vi "Alpha Ver 1.2.vi"() -> ()   [LabVIEW 2015]
uses:
  <instrlib>/Keithley 622x LV 2009/Configure/Source/Typedefs/KE622x -- Current Range.ctl
  <instrlib>/Keithley 622x LV 2009/Configure/Source/Typedefs/KE622x -- Current Ranges.ctl
  <instrlib>/Keithley 622x LV 2009/Typedefs/KE622x -- On Off Control.ctl
  <instrlib>/Keithley 622x LV 2009/Utility/Typedefs/KE622x -- Instrument Type.ctl
  <instrlib>/Keithley 622x LV 2009/Configure/Source/Typedefs/KE622x -- Voltage Limit.ctl
  <instrlib>/Keithley 2000/Public/Configure/Configure DC Volts.vi
  <userlib>/LV-Link3/PolySubVIs/DtCreateAinChan.vi
  <userlib>/LV-Link3/PolySubVIs/DtOLReadMultipleSingle.vi
  <instrlib>/Keithley 2000/Keithley 2000.lvlib
  <instrlib>/Keithley 622x LV 2009/Keithley 622x.lvlib
panel:
  out "DAQ A4":dbl format="%#_13g"
  out "DAQ_clust":T1
  out "DAQ A3":dbl format="%#_13g"
  out "DAQ A2":dbl format="%#_13g"
  out "DAQ A1":dbl format="%#_13g"
  out "Real stop cur":dbl format="%#_13g"
  out "Real start cur":dbl format="%#_13g"
  in  "Stop cur prefix":u16(ring)=2
  in  "Start cur prefix":u16(ring)=2
  out "MULTIPLE GRAPHS":cluster{dbl[], dbl[]}[](graph)
  in  "X-Axis":T2(ring)
  in  "Range":u8(ring)=20 items=["100nV", "200nV", "500nV", "1µV", "2µV", "5µV", "10µV", "20µV", "50µV", "100µV", "200µV", "500µV", "1mV", "2mV", "5mV", "10mV", "20mV", "50mV", "100mV", "200mV", "500mV", "1V"]
  in  "Display Type copy":u16(ring)=3 items=["X %", "Y %", "X Calibrated", "Y Calibrated", "Mag %", "Mag Calibrated", "Phase Degrees", "Ratio", "ADC 1", "ADC 2", "ADC 3", "ADC 4 ", "Noise %", "Noise Calibrated", "Ref Frequency", "", ""]
  out "Units copy":string
  out "Display copy":dbl format="%.3f"
  out "Overload":bool
  out "Display":dbl format="%.3f"
  out "Units":string
  in  "Display Type":u16(ring)=2 items=["X %", "Y %", "X Calibrated", "Y Calibrated", "Mag %", "Mag Calibrated", "Phase Degrees", "Ratio", "ADC 1", "ADC 2", "ADC 3", "ADC 4 ", "Noise %", "Noise Calibrated", "Ref Frequency", "", ""]
  in  "Time Constant":u16(ring) items=["MIN", "1ms", "3ms", "10ms", "30ms", "100ms", "300ms", "1s", "3s", "10s", "30s", "100s", "300s"]
  in  "Slope":u8(ring) items=["6db/octave", "12dB/octave"]
  in  "Dynamic Reserve":u16(ring) items=["High Stability", "Normal", "High Reserve"]
  in  "Auto Sensitivity":bool
  in  "Auto Measure":bool
  out "6221_error_out":errorcluster
  out "2000_error_out":errorcluster
  out "5110_error_out":errorcluster
  out "Input Mode":i32(ring) items=[" Voltage Input (A or A-B) ", "Current Input 10E6 V/A", "Current Input 10E8 V/A"]
  out "5110":refnum<visa-resource-name>
  in  "GPIB Address":i8=11 min=1 max=32 step=1
  out "DAQ A0":dbl format="%#_13g"
  out "2000":dbl format="%#_13g"
  in  "Device":string(combo)
  in  "Number \nof points":i32
  in  "Folder\nprename":string
  out "TIME GRAPH":cluster{dbl[], dbl[]}[](graph)
  out "T0":u32
  out "LIMIT":bool
  out "LIMIT":bool
  out "Error Code":string
  in  "Comments":string
  out "file":refnum<file>
  out "2000":refnum<visa-resource-name>
  out "6221":refnum<visa-resource-name>
  out "Step  (A)":dbl=5e-05 format="%#_3p"
  in  "Stop\ncurrent (A)":dbl=2.0 format="%#_6p"
  in  "Start \ncurrent (A)":dbl=1.0 format="%#_6p"
  in  "Check For SCPI Errors? (T)":bool=TRUE
  out "Interlock Tripped?":bool
  out "Compliance?":bool
  in  "Turn Off Output \nIf Compliance?":bool=TRUE
  in  "Turning ON/OFF\ncurrent output":T3=enum."On"
  in  "Range Selection":T4={"Auto Range?"=TRUE, "Man / Selected\nRange"=enum."2nA"}
  # "FILE CONFIGURATION"
  # "ADMIN PANEL"
  # "KEITHLEY 6221 CONFIGURATION (ADMIN ONLY)"
  # "KEITHLEY DAQ CONFIGURATION (ADMIN ONLY)"
  # "PRINCETON LOCK-IN AMP (ADMIN ONLY)"
  # "I don't know what the hell it is,\njust don't touch it"
  # "SENSITIVITY"
  # "INPUT CONFIGURATION"
  # "READINGS"
  # "START, STOP, STEP, CONFIGURATION"
  # "IF ON"
  # "Output Channels Time - Constant \nSlope & Dynamic Reserve"
  # "Compliance = Limiting output voltage\nThis switch determines if we want to switch \noff the current output if wee exceed compliance"
  # "LOCK-IN READINGS"
  # "RIGHT DISPLAY"
  # "LEFT DISPLAY"
  # "There is a safe switch at \nthe back of the instrument \nThis indicator shows if it is on"
  # "You have hit a damn jackpot \nby exceeding the limited voltage\nCongrats"
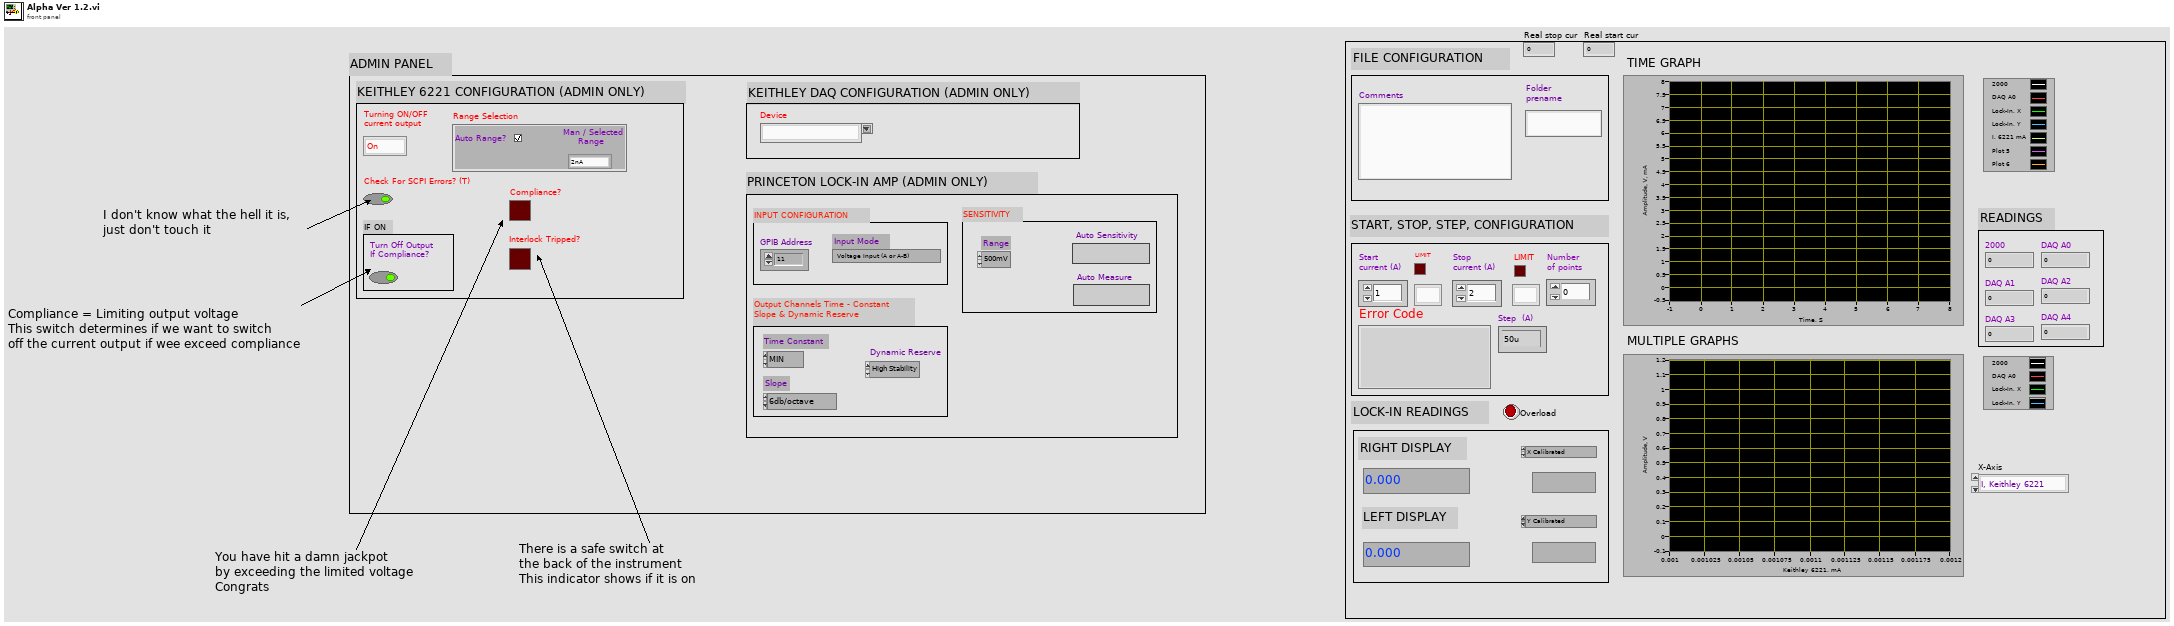
[diagram p1: front panel]
types:
  T1 = cluster{"Task out":i32, "Actual Number of Channels":u32, "error out":errorcluster}
  T2 = enum16{"I, Keithley 6221", "V, Keithley 2000", "V, Keithley DAQ A0", "V, Keithley DAQ A1", "V, Keithley DAQ A2", "V, Keithley DAQ A3", "V, Keithley DAQ A4", "V, Lock-In X", "V, Lock-In Y"}
  T3 = typedef "Keithley 622x.lvlib/KE622x -- On Off Control.ctl" = enum16{"Off", "On"}
  T4 = typedef "Keithley 622x.lvlib/KE622x -- Current Range.ctl" = cluster{"Auto Range?":bool, "Man / Selected\nRange":T5}
  T5 = typedef "Keithley 622x.lvlib/KE622x -- Current Ranges.ctl" = enum16{"2nA", "20nA", "200nA", "2uA", "20uA", "200uA", "2mA", "20mA", "100mA"}
  T6 = typedef "Keithley 622x.lvlib/KE622x -- Instrument Type.ctl" = enum16{"KE6220", "KE6221"}
  T7 = typedef "Keithley 622x.lvlib/KE622x -- Voltage Limit.ctl" = dbl
  T8 = cluster{"Task out":i32, "error out":errorcluster}
  T9 = cluster{dbl, dbl, dbl, dbl, dbl, "Measurement":dbl}
  T10 = cluster{dbl[], dbl[], dbl[], dbl[], dbl[], dbl[], dbl[], dbl[], dbl[], dbl[]}
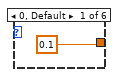
[diagram p2: hidden frame]
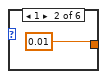
[diagram p3: hidden frame]
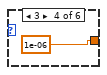
[diagram p4: hidden frame]
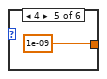
[diagram p5: hidden frame]
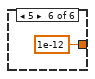
[diagram p6: hidden frame]
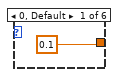
[diagram p7: hidden frame]
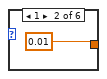
[diagram p8: hidden frame]
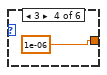
[diagram p9: hidden frame]
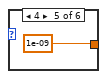
[diagram p10: hidden frame]
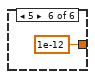
[diagram p11: hidden frame]
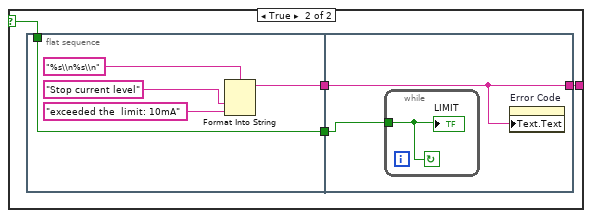
[diagram p12: hidden frame]
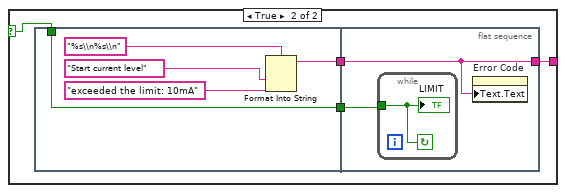
[diagram p13: hidden frame]
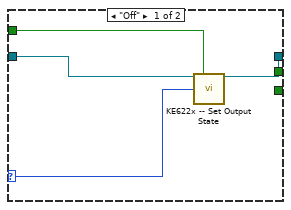
[diagram p14: hidden frame]
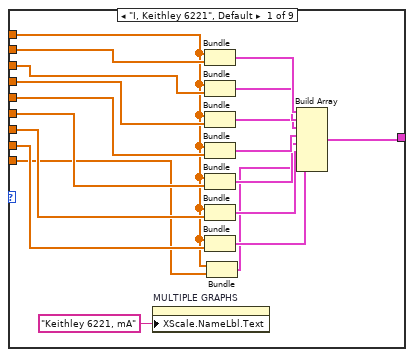
[diagram p15: hidden frame]
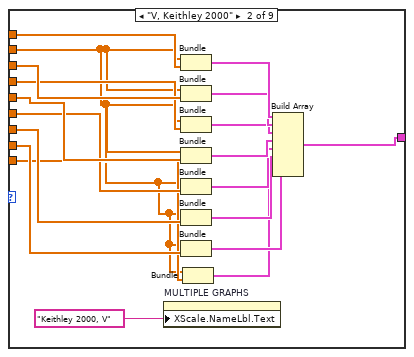
[diagram p16: hidden frame]
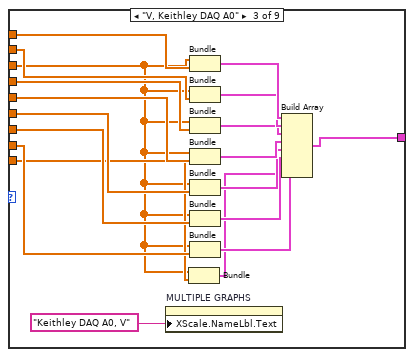
[diagram p17: hidden frame]
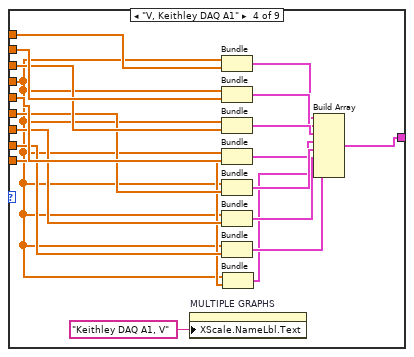
[diagram p18: hidden frame]
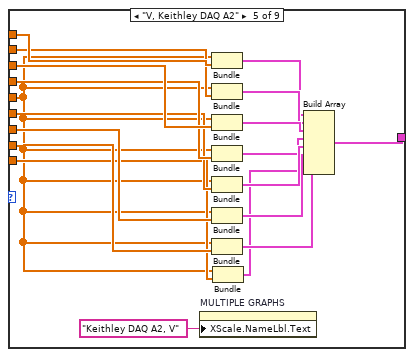
[diagram p19: hidden frame]
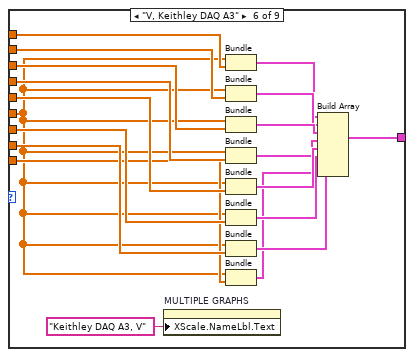
[diagram p20: hidden frame]
diagram:
  n1 = flat-sequence {
    tunnel: [w175] -> w7
    tunnel: [w174] -> w6
    tunnel: [w173] -> w5
    tunnel: [w172] -> w4
    tunnel: [w171] -> w3
    tunnel: [w170] -> w2
    tunnel: [w159] -> w1
    tunnel: w7 -> [w800]
    tunnel: w6 -> [w799]
    tunnel: w5 -> [w798]
    tunnel: w4 -> [w797]
    tunnel: w3 -> [w796]
    tunnel: w2 -> [w795]
    tunnel: w1 -> [w794]
    frame #0 {
      # "File configuration"
      # "Start, Stop, Step"
      # "Time Intit"
      # "Initializing instruments"
      n2 = flat-sequence {
        frame #0 {
          w16 = TRUE  # reset
          w15 = FALSE  # ID query
          # "Initialize Lock-In 5110"
          # "Initialize Keithley 2000"
          # "Initialize Keithley 6221"
          n3 = call <instrlib>:"Initialize.vi"("VISA resource name"=refnum<visa-resource-name> "KEITHLEY_MULTIMETER") -> ("VISA resource name out"=w20:refnum<visa-resource-name>)  [unwired: 17 in, 1 out]
          n4 = call <instrlib>:"Initialize.vi"("VISA resource name"=refnum<visa-resource-name> "KEITHLEY_DC_AC_CURRENT_SOURCE", "Error Queue Option"=enum16{"Clear Error Queue", "Error Query"}."Clear Error Queue", "Instrument Type"=KE622x_--_Instrument_Type."KE6221") -> ("VISA resource name out"=→"6221":refnum<visa-resource-name>, "error out"=→"6221_error_out":errorcluster)  [unwired: 11 in]
          n5 = call "SR51XX Initialize"("VISA session (for class)"=refnum<visa-resource-name> "LOCK_IN_5110_PRINCETON", "Interface"=FALSE, "ID query"=w15, "GPIB Address"="GPIB Address", "reset"=w16) -> ("VISA session"=→"5110":refnum<visa-resource-name>, "error out"=→"5110_error_out":errorcluster)  [unwired: 8 in, 1 out]
          n6 = call-poly <instrlib>:"Configure Measurement.vi"("VISA resource name"=w20) -> ("VISA resource name out"=→"2000":refnum<visa-resource-name>, "error out"=→"2000_error_out":errorcluster)  [unwired: 17 in]
        }
        frame #1 {
          # "Initialize Keithley DAQ \n(getting board name)"
          n7 = call <userlib>:"DtOLGetBoardNames.vi"() -> ("Number of boards"=w25:u32)  [unwired: 9 in, 2 out]
          n8 = Initialize Array("", w25) -> (w27:string[])
          n9 = for {
            N: w25 -> [_]
            shift-right: [w33] -> w30
            shift-left: w27 -> [w34]
            i -> [w32]
            n10 = Add(x=1, y=w32) -> (x+y=w36:i32)
            n11 = call <userlib>:"DtOLGetBoardNames.vi"("Select Board"=w36) -> ("Board Name"=w31:string)  [unwired: 8 in, 2 out]
            n12 = Replace Array Subset(array=w34, new element=w31, index=w32) -> (w33:string[])
          }
          n13 = Index Array(array=w30, index=0) -> (element=w29:string)
          n14 = property on="Device" class="CmbBox"("Strings[]"=w30, "Value"=w29) -> ()  [unwired: 2 in, 2 out]
        }
        frame #2 {
          # "Calculating steps by number\nof points"
          # "Putting in a loop \ninstead of \"STOP\""
          n15 = local read "Real stop cur"() -> (w53:dbl)
          n16 = local read "Real start cur"() -> (w54:dbl)
          n17 = case shown="2" "Start cur prefix" {
            tunnel: [0.1 0.01 0.001 1e-06 1e-09 1e-12] -> w42
            frame 0, Default {
            }
            frame 1 {
            }
            frame 2 {
            }
            frame 3 {
            }
            frame 4 {
            }
            frame 5 {
            }
          }
          n18 = case shown="2" "Stop cur prefix" {
            tunnel: [0.1 0.01 0.001 1e-06 1e-09 1e-12] -> w40
            frame 0, Default {
            }
            frame 1 {
            }
            frame 2 {
            }
            frame 3 {
            }
            frame 4 {
            }
            frame 5 {
            }
          }
          n19 = Subtract(x=w53, y=w54) -> (x-y=w56:dbl)
          n20 = Multiply(x=w42, y="Start \ncurrent (A)") -> (x*y=w38:dbl)
          "Real start cur" <- w38
          n21 = Divide(x=w56, y="Number \nof points") -> (x/y=→"Step  (A)":dbl)
          n22 = Multiply(x=w40, y="Stop\ncurrent (A)") -> (x*y=w37:dbl)
          "Real stop cur" <- w37
          n23 = Greater?(x=w37, y=T7 0.01) -> (0:w48:bool)
          n24 = Greater?(x=w38, y=T7 0.01) -> (0:w47:bool)
          n25 = case shown="False" w48 {
            selector: w48 -> [_ w72]
            tunnel: [w69 w75] -> w50
            frame False {
              n26 = Format Into String(format string="%s\\n", "Start current level is OK" ("false string")) -> (resulting string=w69:string)  [unwired: 2 in, 1 out]
            }
            frame True {
              n27 = flat-sequence {
                tunnel: [w77] -> w74
                tunnel: [w76] -> w73
                tunnel: w72 -> [w76]
                tunnel: [w81] -> w75
                tunnel: w74 -> [w81]
                tunnel: w73 -> [w82]
                frame #0 {
                  n28 = Format Into String(format string="%s\\n%s\\n", "Stop current level" ("String"), "exceeded the  limit: 10mA" ("input 2")) -> (resulting string=w77:string)  [unwired: 2 in, 1 out]
                }
                frame #1 {
                  n29 = while {
                    tunnel: w82 -> [w83]
                    stop <- w83 continue-if-true
                    "LIMIT" <- w83
                  }
                  n30 = property on="Error Code" class="Str"("Text.Text"=w81) -> ()  [unwired: 2 in, 2 out]
                }
              }
            }
          }
          n31 = case shown="False" w47 {
            selector: w47 -> [_ w88]
            tunnel: [w84 w90] -> w49
            frame False {
              n32 = Format Into String(format string="%s\\n", "Start current level is OK" ("false string")) -> (resulting string=w84:string)  [unwired: 2 in, 1 out]
            }
            frame True {
              n33 = flat-sequence {
                tunnel: [w92] -> w89
                tunnel: w88 -> [w91]
                tunnel: [w91] -> w87
                tunnel: [w96] -> w90
                tunnel: w89 -> [w96]
                tunnel: w87 -> [w97]
                frame #0 {
                  n34 = Format Into String(format string="%s\\n%s\\n", "Start current level" ("String"), "exceeded the limit: 10mA" ("input 2")) -> (resulting string=w92:string)  [unwired: 2 in, 1 out]
                }
                frame #1 {
                  n35 = while {
                    tunnel: w97 -> [w98]
                    stop <- w98 continue-if-true
                    "LIMIT" <- w98
                  }
                  n36 = property on="Error Code" class="Str"("Text.Text"=w96) -> ()  [unwired: 2 in, 2 out]
                }
              }
            }
          }
          n37 = Concatenate Strings(w49, w50) -> (→"Error Code":string)
        }
        frame #3 {
          n38 = flat-sequence {
            frame #0 {
              # "Creating folder&file"
              n39 = call "folder_creation.vi"("Name"="Folder\nprename") -> ("String"=w100:string)
              n40 = call "file_creation.vi"("String"=w100) -> ("refnum out"=→"file":refnum<file>)
            }
            frame #1 {
              # "Creating comments"
              n41 = local read "file"() -> (w102:refnum<file>)
              n42 = Format Into String(format string="# %s\\n", initial string=w102, "Comments") -> ()  [unwired: 1 in, 2 out]
            }
            frame #2 {
              # "Writing instr params"
              n43 = local read "5110"() -> (w110:refnum<visa-resource-name>)
              n44 = local read "Real stop cur"() -> (w108:dbl)
              n45 = local read "file"() -> (w105:refnum<file>)
              n46 = local read "Real start cur"() -> (w109:dbl)
              n47 = call "com_inst.vi"("Stop current"=w108, "Start current"=w109, "VISA session (for class)"=w110) -> ("concatenated string"=w106:string)
              n48 = Format Into String(format string="# %s\\n", initial string=w105, w106) -> ()  [unwired: 1 in, 2 out]
            }
            frame #3 {
              # "Adding headlines"
              n49 = local read "file"() -> (w122:refnum<file>)
              n50 = Format Into String(format string="# %-6s  %-12s %-12s %-14s %-12s %-14s %-12s %-14s %-14s%-14s\\n", initial string=w122, "t, ms" ("input 3"), "2000, V" ("input 1"), "DAQ A0, V" ("input 2"), "DAQ A1, V" ("input 2"), "DAQ A2, V" ("input 2"), "DAQ A3, V" ("input 2"), "DAQ A4, V" ("input 2"), "5110_X" ("input 3"), "5110_Y " ("input 3"), "6221, mA" ("input 3")) -> ()  [unwired: 1 in, 2 out]
            }
          }
        }
      }
      n51 = Tick Count (ms)() -> (millisecond timer value=→"T0":u32)
    }
    frame #1 {
      # "Configuring Keithley DAQ just before measuments"
      # "Configuring Keithley 6221 just before measuments"
      n52 = flat-sequence {
        tunnel: [w133] -> w123
        tunnel: [w151] -> _
        tunnel: [w153] -> _
        tunnel: w123 -> [w152]
        frame #0 {
          # "Current range \nselection check"
          # "Checking for compliance\nand interlock errors"
          n53 = local read "6221"() -> (w136:refnum<visa-resource-name>)
          n54 = call <instrlib>:"KE622x -- Set Current Range.vi"("Resource In"=w136, "Current Range In"="Range Selection", "Read Back Set Values? (T)"=FALSE) -> ("Resource Out (dupl)"=w141:refnum<visa-resource-name>)  [unwired: 10 in, 2 out]
          n55 = case shown="\"On\"" "Turning ON/OFF\ncurrent output" {
            selector: "Turning ON/OFF\ncurrent output" -> [w145 _]
            tunnel: [_ w149] -> w139
            tunnel: [_ w148] -> w140
            tunnel: "Check For SCPI Errors? (T)" -> [w144 _]
            tunnel: w141 -> [w142 w147]
            tunnel: [w143 w146] -> w133
            frame "Off" {
              n56 = call <instrlib>:"KE622x -- Set Output State.vi"("Resource In"=w142, "Check For SCPI Errors? (T)"=w144, "Output State"=w145) -> ("Resource Out (dupl)"=w143:refnum<visa-resource-name>)  [unwired: 11 in, 1 out]
            }
            frame "On" {
              n57 = call <instrlib>:"KE622x -- Turn Output On And Check For Errors.vi"("Resource In"=w147, "Turn Off Output If Compliance?"="Turn Off Output \nIf Compliance?") -> ("Resource Out (dupl)"=w146:refnum<visa-resource-name>, "Interlock Tripped?"=w149:bool, "Compliance?"=w148:bool)  [unwired: 10 in, 1 out]
            }
          }
          "Interlock Tripped?" <- w139
          "Compliance?" <- w140
        }
        frame #1 {
          # "Setting start current"
          n58 = local read "Real start cur"() -> (w151:dbl)
          n59 = Wait (ms)(milliseconds to wait=u32 100) -> ()  [unwired: 1 out]
          n60 = call <instrlib>:"KE622x -- Set Current Level.vi"("Resource In"=w152, "Current Level (A) In"=w151) -> ("Resource Out (dupl)"=w153:refnum<visa-resource-name>)  [unwired: 12 in, 1 out]
        }
      }
      n61 = flat-sequence {
        frame #0 {
          w128 = 100 items=["SingleEnded"=100, "Differential"=101] ("Channel Type")
          # "Configure the input channel"
          n62 = call-poly <userlib>:"DtOLCreateTask.vi"("Channel Type"=w128, "Range Min"=-10.0, "Range Max"=10.0, "Board Name"="Device", "Channel"="0:4" ("Channels")) -> ("Task out"=w127:i32, "Actual Number of Channels"=w126:u32, "error out"=w125:errorcluster)  [unwired: 8 in]
          n63 = Bundle("Task out"=w127, "Actual Number of Channels"=w126, "error out"=w125) -> (→"DAQ_clust":T1)  [unwired: 1 in]
        }
      }
    }
    frame #2 {
      n64 = local read "5110"() -> (w166:refnum<visa-resource-name>)
      n65 = local read "2000"() -> (w165:refnum<visa-resource-name>)
      n66 = local read "6221"() -> (w164:refnum<visa-resource-name>)
      n67 = local read "5110_error_out"() -> (w163:errorcluster)
      n68 = local read "6221_error_out"() -> (w162:errorcluster)
      n69 = local read "2000_error_out"() -> (w161:errorcluster)
      n70 = local read "DAQ_clust"() -> (w160:T1)
      n71 = while {
        shift-right: [w252] -> _
        shift-left: dbl[] [] -> [w406]
        shift-right: [w253] -> _
        shift-left: i32[] [] -> [w405]
        tunnel: w165 -> [w403]
        tunnel: w164 -> [w402]
        shift-right: [w184] -> _
        shift-left: dbl[] [] -> [w395]
        tunnel: [w394] -> w175
        tunnel: [w393] -> w174
        tunnel: [w391] -> w173
        tunnel: [w388] -> w172
        tunnel: w166 -> [w385]
        tunnel: w163 -> [w384]
        tunnel: w162 -> [w376]
        tunnel: w161 -> [w375]
        tunnel: [w326] -> w171
        tunnel: [w323] -> w170
        shift-right: [w186] -> _
        shift-left: dbl[] [] -> [w322]
        shift-right: [w187] -> _
        shift-left: dbl[] [] -> [w321]
        shift-right: [w254] -> _
        shift-left: dbl[] [] -> [w318]
        tunnel: w160 -> [w275]
        tunnel: [w274] -> w159
        shift-right: [w251] -> _
        shift-left: dbl[] [] -> [w273]
        shift-right: [w250] -> _
        shift-left: dbl[] [] -> [w272]
        shift-right: [w249] -> _
        shift-left: dbl[] [] -> [w271]
        shift-right: [w185] -> _
        shift-left: dbl[] [] -> [w190]
        i -> [w377]
        stop <- w396 stop-if-true
        # "V, DAQ A4"
        # "V, DAQ A3"
        # "V, DAQ A2"
        # "V, DAQ A1"
        # "Y-V, 5110"
        # "X-V, 5110"
        # "I, 6221"
        # "Config delay"
        # "Control subVI 5110"
        # "Read config 5110"
        # "Measurement config 5110"
        # "Time config 5110"
        # "Configuring Right Display 5110"
        # "Configuring Left Display 5110"
        # "Setting 6221 current"
        # "Delay before measuremens"
        # "Getting the data from DAQ and 2000"
        # "Changing input current"
        # "Time"
        # "V, DAQ A0"
        # "V, 2000"
        n72 = local read "T0"() -> (w404:u32)
        n73 = Quotient & Remainder(x=w377, y=10) -> (floor(x/y)=w382:i32)  [unwired: 1 out]
        n74 = Equal?(x=0, y=w377) -> (x = y?=w379:bool)
        n75 = Subtract(x=w366, y=w404) -> (x-y=w286:u32)
        n76 = Equal?(x=1, y=w382) -> (x = y?=w378:bool)
        n77 = flat-sequence {
          tunnel: w403 -> [w588]
          tunnel: [w588] -> w317
          tunnel: w402 -> [w587]
          tunnel: [w587] -> w315
          tunnel: w385 -> [w585]
          tunnel: [w585] -> w313
          tunnel: [w584] -> w311
          tunnel: w384 -> [w584]
          tunnel: w379 -> [w583]
          tunnel: [w583] -> w309
          tunnel: w378 -> [w582]
          tunnel: [w582] -> w307
          tunnel: w376 -> [w581]
          tunnel: [w581] -> w305
          tunnel: w375 -> [w580]
          tunnel: [w580] -> w303
          tunnel: [w579] -> w366
          tunnel: [w578] -> w276
          tunnel: w275 -> [w578]
          tunnel: w317 -> [w603]
          tunnel: [w603] -> w316
          tunnel: w315 -> [w602]
          tunnel: [w602] -> w314
          tunnel: w313 -> [w601]
          tunnel: [w601] -> w312
          tunnel: w311 -> [w600]
          tunnel: [w600] -> w310
          tunnel: w309 -> [w599]
          tunnel: [w599] -> w308
          tunnel: w307 -> [w598]
          tunnel: [w598] -> w306
          tunnel: w305 -> [w597]
          tunnel: [w597] -> w304
          tunnel: w303 -> [w596]
          tunnel: [w596] -> w302
          tunnel: [w589] -> w277
          tunnel: w276 -> [w589]
          tunnel: w316 -> [w616]
          tunnel: [w616] -> w365
          tunnel: w314 -> [w615]
          tunnel: [w615] -> w364
          tunnel: w312 -> [w614]
          tunnel: w310 -> [w611]
          tunnel: [w610] -> w363
          tunnel: [w609] -> w362
          tunnel: w308 -> [w608]
          tunnel: [w608] -> w361
          tunnel: w306 -> [w607]
          tunnel: w304 -> [w606]
          tunnel: [w606] -> w360
          tunnel: w302 -> [w605]
          tunnel: [w605] -> w359
          tunnel: [w604] -> w278
          tunnel: w277 -> [w604]
          tunnel: w365 -> [w641]
          tunnel: [w641] -> w358
          tunnel: w364 -> [w640]
          tunnel: [w640] -> w357
          tunnel: w363 -> [w637]
          tunnel: [w636] -> w356
          tunnel: w362 -> [w635]
          tunnel: [w634] -> w355
          tunnel: w361 -> [w632]
          tunnel: [w632] -> w354
          tunnel: w360 -> [w639]
          tunnel: [w639] -> w353
          tunnel: w359 -> [w638]
          tunnel: [w638] -> w352
          tunnel: ["Auto Measure"] -> w351
          tunnel: ["Auto Sensitivity"] -> w350
          tunnel: [w627] -> w349
          tunnel: [w624] -> w279
          tunnel: w278 -> [w624]
          tunnel: w358 -> [w660]
          tunnel: [w660] -> w301
          tunnel: w357 -> [w659]
          tunnel: [w659] -> w300
          tunnel: w356 -> [w652]
          tunnel: w355 -> [w650]
          tunnel: [w649] -> w299
          tunnel: w354 -> [w656]
          tunnel: [w656] -> w298
          tunnel: w353 -> [w658]
          tunnel: [w658] -> w297
          tunnel: w352 -> [w657]
          tunnel: [w657] -> w296
          tunnel: w351 -> [w654]
          tunnel: [w654] -> w295
          tunnel: w350 -> [w655]
          tunnel: [w655] -> w294
          tunnel: w349 -> [w645]
          tunnel: [w645] -> w293
          tunnel: [w651] -> w292
          tunnel: ["Time Constant"] -> w291
          tunnel: ["Slope"] -> w290
          tunnel: [w642] -> w280
          tunnel: w279 -> [w642]
          tunnel: [w684] -> w348
          tunnel: [w683] -> w347
          tunnel: [w669] -> w346
          tunnel: [w682] -> w345
          tunnel: [w681] -> w344
          tunnel: [w680] -> w343
          tunnel: [w679] -> w342
          tunnel: [w678] -> w341
          tunnel: [w671] -> w340
          tunnel: [w674] -> w339
          tunnel: [w672] -> w338
          tunnel: [w677] -> w337
          tunnel: [w662] -> w267
          tunnel: w290 -> [w677]
          tunnel: w291 -> [w672]
          tunnel: w292 -> [w675]
          tunnel: w293 -> [w671]
          tunnel: w294 -> [w678]
          tunnel: w295 -> [w679]
          tunnel: w296 -> [w680]
          tunnel: w297 -> [w681]
          tunnel: w298 -> [w682]
          tunnel: w299 -> [w670]
          tunnel: w300 -> [w683]
          tunnel: w301 -> [w684]
          tunnel: [w661] -> w281
          tunnel: w280 -> [w661]
          tunnel: w348 -> [w708]
          tunnel: [w708] -> w336
          tunnel: w347 -> [w707]
          tunnel: [w707] -> w335
          tunnel: w346 -> [w694]
          tunnel: w345 -> [w706]
          tunnel: [w706] -> w334
          tunnel: w344 -> [w705]
          tunnel: [w705] -> w333
          tunnel: w343 -> [w704]
          tunnel: [w704] -> w332
          tunnel: w342 -> [w703]
          tunnel: [w703] -> w331
          tunnel: w341 -> [w702]
          tunnel: [w702] -> w330
          tunnel: w340 -> [w695]
          tunnel: w339 -> [w692]
          tunnel: [w691] -> w329
          tunnel: w338 -> [w696]
          tunnel: w337 -> [w697]
          tunnel: [w693] -> w328
          tunnel: [w690] -> w327
          tunnel: [w686] -> w266
          tunnel: [w685] -> w282
          tunnel: w281 -> [w685]
          tunnel: [w712] -> w400
          tunnel: w377 -> [w720]
          tunnel: [w716] -> w396
          tunnel: [w710] -> w398
          tunnel: [w718] -> w397
          tunnel: [w715] -> w374
          tunnel: [w714] -> w373
          tunnel: [w713] -> w372
          tunnel: [w711] -> w371
          tunnel: [w710] -> w268
          tunnel: w327 -> [_]
          tunnel: w328 -> [w713]
          tunnel: w329 -> [w711]
          tunnel: w330 -> [_]
          tunnel: w331 -> [_]
          tunnel: w332 -> [w715]
          tunnel: w333 -> [w714]
          tunnel: w334 -> [_]
          tunnel: w335 -> [w718]
          tunnel: w336 -> [w712]
          tunnel: [w709] -> w283
          tunnel: w282 -> [w709]
          tunnel: w400 -> [w732]
          tunnel: [w732] -> w399
          tunnel: w398 -> [w731]
          tunnel: w397 -> [w730]
          tunnel: [w729] -> w392
          tunnel: [w728] -> w389
          tunnel: w374 -> [w726]
          tunnel: w373 -> [w727]
          tunnel: w372 -> [w724]
          tunnel: w371 -> [w725]
          tunnel: [w726] -> w370
          tunnel: [w725] -> w367
          tunnel: [w724] -> w324
          tunnel: [w723] -> w284
          tunnel: w283 -> [w723]
          tunnel: w399 -> [w740]
          tunnel: [w740] -> w401
          tunnel: w392 -> [w738]
          tunnel: [w738] -> w390
          tunnel: w389 -> [w737]
          tunnel: [w737] -> w387
          tunnel: w370 -> [w736]
          tunnel: [w736] -> w369
          tunnel: [w735] -> w368
          tunnel: w367 -> [w735]
          tunnel: [w734] -> w325
          tunnel: w324 -> [w734]
          tunnel: [w733] -> w285
          tunnel: w284 -> [w733]
          tunnel: [w777] -> w218
          tunnel: [w744] -> w217
          tunnel: [w776] -> w216
          tunnel: [w775] -> w215
          tunnel: [w774] -> w214
          tunnel: [w773] -> w213
          tunnel: [w745] -> w212
          tunnel: [w777] -> w211
          tunnel: [w772] -> w210
          tunnel: [w771] -> w209
          tunnel: [w770] -> w208
          tunnel: w285 -> [w767]
          tunnel: w325 -> [w771]
          tunnel: w368 -> [w772]
          tunnel: w369 -> [w768]
          tunnel: w387 -> [w773]
          tunnel: w390 -> [w774]
          tunnel: w401 -> [w769]
          tunnel: [w743] -> w207
          tunnel: [w742] -> w206
          tunnel: [w741] -> w205
          tunnel: [w781] -> w274
          tunnel: [w782] -> w323
          tunnel: [w783] -> w326
          tunnel: [w784] -> w386
          tunnel: [w785] -> w204
          tunnel: [w786] -> w388
          tunnel: [w787] -> w391
          tunnel: [w788] -> w393
          tunnel: [w789] -> w394
          tunnel: [w790] -> w203
          tunnel: [w791] -> w193
          tunnel: w218 -> [w791]
          tunnel: w217 -> [w790]
          tunnel: w216 -> [w789]
          tunnel: w215 -> [w788]
          tunnel: w214 -> [w787]
          tunnel: w213 -> [w786]
          tunnel: w212 -> [w785]
          tunnel: w211 -> [w784]
          tunnel: w210 -> [w783]
          tunnel: w209 -> [w782]
          tunnel: w208 -> [w781]
          tunnel: [w780] -> w202
          tunnel: w207 -> [w780]
          tunnel: [w779] -> w201
          tunnel: w206 -> [w779]
          tunnel: w205 -> [w778]
          tunnel: [w778] -> w194
          frame #0 {
            n78 = Wait Until Next ms Multiple(millisecond multiple=u32 500) -> (millisecond timer value=w579:u32)
          }
          frame #1 {
            n79 = control-ref of="Range"() -> (w595:refnum<vi>)
            n80 = control-ref of="Auto Sensitivity"() -> (w594:refnum<vi>)
            n81 = control-ref of="Auto Measure"() -> (w593:refnum<vi>)
            n82 = control-ref of="Time Constant"() -> (w590:refnum<vi>)
            n83 = control-ref of="Slope"() -> (w591:refnum<vi>)
            n84 = control-ref of="Dynamic Reserve"() -> (w592:refnum<vi>)
            n85 = call "cont_ver_1.0.vi"("Dynamic Reserve"=w592, "Slope"=w591, "Time Constant"=w590, "Auto Measure"=w593, "Auto Sensitivity"=w594, "Range"=w595) -> ()
          }
          frame #2 {
            n86 = case shown="False" w607 {
              tunnel: w614 -> [w618 w623]
              tunnel: [w617 w621] -> w613
              tunnel: [w618 w620] -> w612
              tunnel: w611 -> [w617 w619]
              frame False {
              }
              frame True {
                n87 = call "SR51XX Read Preamp Input Mode"("VISA session (for class)"=w623, "error in (no error)"=w619) -> ("VISA session"=w620:refnum<visa-resource-name>, "Input Mode"=w622:i32, "error out"=w621:errorcluster)  [unwired: 15 in]
                n88 = local write "Input Mode"(w622) -> ()
              }
            }
            n89 = call "SR51XX Configure Signal Channel Input"("VISA session (for class)"=w612, "error in (no error)"=w613, "Update"=w608) -> ("VISA session"=w610:refnum<visa-resource-name>, "error out"=w609:errorcluster)  [unwired: 15 in]
          }
          frame #3 {
            n90 = local read "Input Mode"() -> (w633:i32)
            n91 = call "SR51XX Configure Sensitivity"("VISA session (for class)"=w637, "Input Mode"=w633, "Range"="Range", "error in (no error)"=w635, "Auto Sensitivity"="Auto Sensitivity", "Auto Measure"="Auto Measure", "Update"=w632) -> ("Range Annotations Out[]"=w625:string[], "VISA session"=w636:refnum<visa-resource-name>, "Auto Sensitivity out"=w629:bool, "Auto Measure out"=w628:bool, "Range Out"=w627:u8, "error out"=w634:errorcluster)  [unwired: 7 in]
            n92 = property on="Range" class="Ring (strict)"("Strings []"=w625) -> ()  [unwired: 2 in, 2 out]
            n93 = local write "Auto Sensitivity"(w629) -> ()
            n94 = local write "Auto Measure"(w628) -> ()
            n95 = local write "Range"(w627) -> ()
          }
          frame #4 {
            n96 = Or(x=w655, y=w654) -> (x .or. y?=w653:bool)
            n97 = call "SR51XX Configure Output Channels - Slope, TC and Dyn Reserve"("VISA session (for class)"=w652, "Time Constant"="Time Constant", "Slope"="Slope", "Check TC"=w653, "Dynamic Reserve"="Dynamic Reserve", "error in (no error)"=w650, "Range"=w645, "Update"=w656) -> ("VISA session"=w651:refnum<visa-resource-name>, "Slope Out"=w646:u8, "Time Constant Out"=w647:u16, "error out"=w649:errorcluster)  [unwired: 8 in]
            n98 = local write "Slope"(w646) -> ()
            n99 = local write "Time Constant"(w647) -> ()
          }
          frame #5 {
            n100 = local read "Input Mode"() -> (w676:i32)
            n101 = call "SR5110 Read Output"("VISA session (for class)"=w675, "Input Mode"=w676, "Time Constant"=w672, "Display Type"="Display Type", "Range"=w671, "error in (no error)"=w670, "Slope"=w677) -> ("Units"=w664:string, "Display Precision"=w668:i32, "Display"=w663:dbl, "VISA session"=w674:refnum<visa-resource-name>, "Available Display Types Out"=w667:string[], "Overload"=→"Overload":bool, "error out"=w669:errorcluster)  [unwired: 4 in, 2 out]
            "Units" <- w664
            "Display" <- w663
            n102 = property on="Display Type" class="Ring (strict)"("Strings []"=w667) -> ()  [unwired: 2 in, 2 out]
            n103 = property on="Display" class="DigNum (strict)"("Precision"=w668) -> ()  [unwired: 2 in, 2 out]
            n104 = call "pref_to_num.vi"("string"=w664) -> ("Numeric"=w665:dbl)
            n105 = Multiply(x=w665, y=w663) -> (x*y=w662:dbl)
          }
          frame #6 {
            n106 = local read "Input Mode"() -> (w701:i32)
            n107 = call "SR5110 Read Output"("VISA session (for class)"=w692, "Input Mode"=w701, "Time Constant"=w696, "Display Type"="Display Type copy", "Range"=w695, "error in (no error)"=w694, "Slope"=w697) -> ("Units"=w689:string, "Display Precision"=w698:i32, "Display"=w688:dbl, "VISA session"=w691:refnum<visa-resource-name>, "Reference Unlock"=w690:bool, "Available Display Types Out"=w699:string[], "error out"=w693:errorcluster)  [unwired: 4 in, 2 out]
            "Display copy" <- w688
            "Units copy" <- w689
            n108 = property on="Display Type copy" class="Ring (strict)"("Strings []"=w699) -> ()  [unwired: 2 in, 2 out]
            n109 = property on="Display copy" class="DigNum (strict)"("Precision"=w698) -> ()  [unwired: 2 in, 2 out]
            n110 = call "pref_to_num.vi"("string"=w689) -> ("Numeric"=w687:dbl)
            n111 = Multiply(x=w687, y=w688) -> (x*y=w686:dbl)
          }
          frame #7 {
            n112 = local read "Step  (A)"() -> (w721:dbl)
            n113 = local read "Real start cur"() -> (w722:dbl)
            n114 = Multiply(x=w721, y=w720) -> (x*y=w719:dbl)
            n115 = Add(x=w722, y=w719) -> (x+y=w710:dbl)
            n116 = local read "Real stop cur"() -> (w717:dbl)
            n117 = Greater Or Equal?(x=w710, y=w717) -> (x >= y?=w716:bool)
          }
          frame #8 {
            n118 = call <instrlib>:"KE622x -- Set Current Level.vi"("Resource In"=w730, "Current Level (A) In"=w731, "error in (no error)"=w727) -> ("Resource Out (dupl)"=w728:refnum<visa-resource-name>, "error out"=w729:errorcluster)  [unwired: 11 in]
          }
          frame #9 {
            n119 = Wait Until Next ms Multiple(millisecond multiple=u32 50) -> ()  [unwired: 1 out]
          }
          frame #10 {
            n120 = Unbundle(w767) -> ("Task out"=w766:i32, "Actual Number of Channels"=w764:u32, "error out"=w765:errorcluster)
            n121 = call <instrlib>:"Data Read Single.vi"("VISA resource name"=w769, "error in (no error)"=w768) -> ("VISA resource name out"=w775:refnum<visa-resource-name>, "Measurement"=w777:dbl, "error out"=w776:errorcluster)  [unwired: 13 in, 2 out]
            n122 = call-poly <userlib>:"DtOLRead.vi"("Number Chan to Read"=w764, "error in (no error)"=w765, "Task in"=w766) -> ("error out"=w762:errorcluster, "2D Data out"=w761:dbl[][], "Task out"=w763:i32)  [unwired: 4 in, 2 out]
            n123 = Index Array(array=w761, index (row) #1=0 ("index (row)"), index (row) #2=1 ("index (row)"), index (row) #3=2 ("index (row)"), index (row) #4=3 ("index (row)"), index (row) #5=4 ("index (row)")) -> (element #1=w760:dbl[], element #2=w754:dbl[], element #3=w753:dbl[], element #4=w752:dbl[], element #5=w751:dbl[])  [unwired: 5 in]
            n124 = Index Array(array=w751, index=0) -> (element=w741:dbl)
            n125 = Index Array(array=w760, index=0) -> (element=w745:dbl)
            n126 = Index Array(array=w754, index=0) -> (element=w744:dbl)
            n127 = Index Array(array=w753, index=0) -> (element=w743:dbl)
            n128 = Index Array(array=w752, index=0) -> (element=w742:dbl)
            n129 = Bundle("Task out"=w763, "error out"=w762) -> (w770:T8)  [unwired: 1 in]
          }
          frame #11 {
          }
        }
        n130 = Divide(x=w286, y=u32 1000) -> (x/y=w287:dbl)
        n131 = Build Array (concatenate)(w405, w287) -> (w260:dbl[])
        n132 = local read "file"() -> (w289:refnum<file>)
        n133 = Bundle(w268, w267, w266) -> (w265:cluster{dbl, dbl, dbl})  [unwired: 1 in]
        n134 = Unbundle(w265) -> (w264:dbl, w263:dbl, w262:dbl)
        n135 = Build Array (concatenate)(w322, w263) -> (w192:dbl[])
        n136 = Build Array (concatenate)(w321, w262) -> (w191:dbl[])
        n137 = Build Array (concatenate)(w318, w264) -> (w261:dbl[])
        n138 = Bundle(w204, w203, w202, w201, w194, "Measurement"=w193) -> (w221:T9)  [unwired: 1 in]
        n139 = Unbundle(w221) -> (w269:dbl, w200:dbl, w199:dbl, w198:dbl, w270:dbl, "Measurement"=w189:dbl)
        n140 = Unbundle(w221) -> (w219:dbl, w197:dbl, w196:dbl, w195:dbl, w220:dbl, "Measurement"=w179:dbl)
        n141 = Build Array (concatenate)(w406, w270) -> (w259:dbl[])
        n142 = Build Array (concatenate)(w273, w269) -> (w258:dbl[])
        n143 = Build Array (concatenate)(w272, w200) -> (w257:dbl[])
        n144 = Build Array (concatenate)(w395, w198) -> (w255:dbl[])
        n145 = Build Array (concatenate)(w190, w189) -> (w188:dbl[])
        n146 = Build Array (concatenate)(w271, w199) -> (w256:dbl[])
        n147 = Format Into String(format string="%08d  %8.2e %12g %14.5e %12.4e %12.4e  %12.4e\\n", initial string=w289, w286, w220, w219, w197, w196, w195, w179) -> ()  [unwired: 1 in, 2 out]
        n148 = Bundle(w261, w260, w259, w258, w257, w256, w255, w188, w192, w191) -> (w231:T10)  [unwired: 1 in]
        n149 = Unbundle(w231) -> (w241:dbl[], w182:dbl[], w248:dbl[], w247:dbl[], w246:dbl[], w245:dbl[], w244:dbl[], w243:dbl[], w242:dbl[], w183:dbl[])
        n150 = Bundle(w182, w248) -> (w240:cluster{dbl[], dbl[]})  [unwired: 1 in]
        n151 = Bundle(w182, w247) -> (w239:cluster{dbl[], dbl[]})  [unwired: 1 in]
        n152 = Bundle(w182, w246) -> (w238:cluster{dbl[], dbl[]})  [unwired: 1 in]
        n153 = Bundle(w182, w245) -> (w237:cluster{dbl[], dbl[]})  [unwired: 1 in]
        n154 = Bundle(w182, w244) -> (w236:cluster{dbl[], dbl[]})  [unwired: 1 in]
        n155 = Bundle(w182, w243) -> (w235:cluster{dbl[], dbl[]})  [unwired: 1 in]
        n156 = Bundle(w182, w242) -> (w234:cluster{dbl[], dbl[]})  [unwired: 1 in]
        n157 = Bundle(w182, w241) -> (w233:cluster{dbl[], dbl[]})  [unwired: 1 in]
        n158 = Bundle(w183, w182) -> (w181:cluster{dbl[], dbl[]})  [unwired: 1 in]
        n159 = Build Array(w240, w239, w238, w237, w236, w235, w234, w233, w181) -> (→"TIME GRAPH":cluster{dbl[], dbl[]}[])
        n160 = Unbundle(w231) -> (w230:dbl[], w229:dbl[], w228:dbl[], w227:dbl[], w226:dbl[], w225:dbl[], w224:dbl[], w223:dbl[], w180:dbl[])  [unwired: 1 out]
        n161 = case shown="\"V, Lock-In X\"" "X-Axis" {
          tunnel: [w410 w436 w455 w467 w493 w512 w531 w540 w559] -> w222
          tunnel: w230 -> [w407 w435 w454 w474 w492 w511 w529 w548 w567]
          tunnel: w229 -> [w424 w426 w453 w473 w491 w510 w528 w547 w566]
          tunnel: w228 -> [w423 w434 w445 w472 w490 w509 w527 w546 w565]
          tunnel: w227 -> [w422 w433 w452 w464 w489 w508 w526 w545 w564]
          tunnel: w226 -> [w421 w432 w451 w471 w483 w507 w525 w544 w563]
          tunnel: w225 -> [w420 w431 w450 w470 w488 w502 w524 w543 w562]
          tunnel: w224 -> [w419 w430 w449 w469 w487 w506 w530 w542 w561]
          tunnel: w223 -> [w418 w429 w448 w468 w486 w505 w523 w549 w560]
          tunnel: w180 -> [w408 w427 w446 w465 w484 w503 w522 w541 w568]
          frame "I, Keithley 6221", Default {
            n162 = property on="MULTIPLE GRAPHS" class="XYGraph (strict)"("XScale.NameLbl.Text"="Keithley 6221, mA" ("X Scale.Name Label.Text")) -> ()  [unwired: 2 in, 2 out]
            n163 = Bundle(w407, w424) -> (w417:cluster{dbl[], dbl[]})  [unwired: 1 in]
            n164 = Bundle(w407, w423) -> (w416:cluster{dbl[], dbl[]})  [unwired: 1 in]
            n165 = Bundle(w407, w422) -> (w415:cluster{dbl[], dbl[]})  [unwired: 1 in]
            n166 = Bundle(w407, w421) -> (w414:cluster{dbl[], dbl[]})  [unwired: 1 in]
            n167 = Bundle(w407, w420) -> (w413:cluster{dbl[], dbl[]})  [unwired: 1 in]
            n168 = Bundle(w407, w419) -> (w412:cluster{dbl[], dbl[]})  [unwired: 1 in]
            n169 = Bundle(w407, w418) -> (w411:cluster{dbl[], dbl[]})  [unwired: 1 in]
            n170 = Bundle(w407, w408) -> (w409:cluster{dbl[], dbl[]})  [unwired: 1 in]
            n171 = Build Array(w417, w416, w415, w414, w413, w412, w411, w409) -> (w410:cluster{dbl[], dbl[]}[])
          }
          frame "V, Keithley 2000" {
            n172 = property on="MULTIPLE GRAPHS" class="XYGraph (strict)"("XScale.NameLbl.Text"="Keithley 2000, V" ("X Scale.Name Label.Text")) -> ()  [unwired: 2 in, 2 out]
            n173 = Bundle(w426, w435) -> (w443:cluster{dbl[], dbl[]})  [unwired: 1 in]
            n174 = Bundle(w426, w434) -> (w442:cluster{dbl[], dbl[]})  [unwired: 1 in]
            n175 = Bundle(w426, w433) -> (w441:cluster{dbl[], dbl[]})  [unwired: 1 in]
            n176 = Bundle(w426, w432) -> (w440:cluster{dbl[], dbl[]})  [unwired: 1 in]
            n177 = Bundle(w426, w431) -> (w439:cluster{dbl[], dbl[]})  [unwired: 1 in]
            n178 = Bundle(w426, w430) -> (w438:cluster{dbl[], dbl[]})  [unwired: 1 in]
            n179 = Bundle(w426, w429) -> (w437:cluster{dbl[], dbl[]})  [unwired: 1 in]
            n180 = Bundle(w426, w427) -> (w428:cluster{dbl[], dbl[]})  [unwired: 1 in]
            n181 = Build Array(w443, w442, w441, w440, w439, w438, w437, w428) -> (w436:cluster{dbl[], dbl[]}[])
          }
          frame "V, Keithley DAQ A0" {
            n182 = property on="MULTIPLE GRAPHS" class="XYGraph (strict)"("XScale.NameLbl.Text"="Keithley DAQ A0, V" ("X Scale.Name Label.Text")) -> ()  [unwired: 2 in, 2 out]
            n183 = Bundle(w445, w446) -> (w447:cluster{dbl[], dbl[]})  [unwired: 1 in]
            n184 = Bundle(w445, w454) -> (w462:cluster{dbl[], dbl[]})  [unwired: 1 in]
            n185 = Bundle(w445, w453) -> (w461:cluster{dbl[], dbl[]})  [unwired: 1 in]
            n186 = Bundle(w445, w452) -> (w460:cluster{dbl[], dbl[]})  [unwired: 1 in]
            n187 = Bundle(w445, w451) -> (w459:cluster{dbl[], dbl[]})  [unwired: 1 in]
            n188 = Bundle(w445, w450) -> (w458:cluster{dbl[], dbl[]})  [unwired: 1 in]
            n189 = Bundle(w445, w449) -> (w457:cluster{dbl[], dbl[]})  [unwired: 1 in]
            n190 = Bundle(w445, w448) -> (w456:cluster{dbl[], dbl[]})  [unwired: 1 in]
            n191 = Build Array(w462, w461, w460, w459, w458, w457, w456, w447) -> (w455:cluster{dbl[], dbl[]}[])
          }
          frame "V, Keithley DAQ A1" {
            n192 = property on="MULTIPLE GRAPHS" class="XYGraph (strict)"("XScale.NameLbl.Text"="Keithley DAQ A1, V" ("X Scale.Name Label.Text")) -> ()  [unwired: 2 in, 2 out]
            n193 = Bundle(w464, w474) -> (w476:cluster{dbl[], dbl[]})  [unwired: 1 in]
            n194 = Bundle(w464, w473) -> (w477:cluster{dbl[], dbl[]})  [unwired: 1 in]
            n195 = Bundle(w464, w472) -> (w478:cluster{dbl[], dbl[]})  [unwired: 1 in]
            n196 = Bundle(w464, w471) -> (w479:cluster{dbl[], dbl[]})  [unwired: 1 in]
            n197 = Bundle(w464, w470) -> (w480:cluster{dbl[], dbl[]})  [unwired: 1 in]
            n198 = Bundle(w464, w469) -> (w481:cluster{dbl[], dbl[]})  [unwired: 1 in]
            n199 = Bundle(w464, w468) -> (w482:cluster{dbl[], dbl[]})  [unwired: 1 in]
            n200 = Bundle(w464, w465) -> (w466:cluster{dbl[], dbl[]})  [unwired: 1 in]
            n201 = Build Array(w476, w477, w478, w479, w480, w481, w482, w466) -> (w467:cluster{dbl[], dbl[]}[])
          }
          frame "V, Keithley DAQ A2" {
            n202 = property on="MULTIPLE GRAPHS" class="XYGraph (strict)"("XScale.NameLbl.Text"="Keithley DAQ A2, V" ("X Scale.Name Label.Text")) -> ()  [unwired: 2 in, 2 out]
            n203 = Bundle(w483, w492) -> (w494:cluster{dbl[], dbl[]})  [unwired: 1 in]
            n204 = Bundle(w483, w491) -> (w495:cluster{dbl[], dbl[]})  [unwired: 1 in]
            n205 = Bundle(w483, w490) -> (w496:cluster{dbl[], dbl[]})  [unwired: 1 in]
            n206 = Bundle(w483, w489) -> (w497:cluster{dbl[], dbl[]})  [unwired: 1 in]
            n207 = Bundle(w483, w488) -> (w498:cluster{dbl[], dbl[]})  [unwired: 1 in]
            n208 = Bundle(w483, w487) -> (w499:cluster{dbl[], dbl[]})  [unwired: 1 in]
            n209 = Bundle(w483, w486) -> (w500:cluster{dbl[], dbl[]})  [unwired: 1 in]
            n210 = Bundle(w483, w484) -> (w485:cluster{dbl[], dbl[]})  [unwired: 1 in]
            n211 = Build Array(w494, w495, w496, w497, w498, w499, w500, w485) -> (w493:cluster{dbl[], dbl[]}[])
          }
          frame "V, Keithley DAQ A3" {
            n212 = property on="MULTIPLE GRAPHS" class="XYGraph (strict)"("XScale.NameLbl.Text"="Keithley DAQ A3, V" ("X Scale.Name Label.Text")) -> ()  [unwired: 2 in, 2 out]
            n213 = Bundle(w502, w511) -> (w513:cluster{dbl[], dbl[]})  [unwired: 1 in]
            n214 = Bundle(w502, w510) -> (w514:cluster{dbl[], dbl[]})  [unwired: 1 in]
            n215 = Bundle(w502, w509) -> (w515:cluster{dbl[], dbl[]})  [unwired: 1 in]
            n216 = Bundle(w502, w508) -> (w516:cluster{dbl[], dbl[]})  [unwired: 1 in]
            n217 = Bundle(w502, w507) -> (w517:cluster{dbl[], dbl[]})  [unwired: 1 in]
            n218 = Bundle(w502, w506) -> (w518:cluster{dbl[], dbl[]})  [unwired: 1 in]
            n219 = Bundle(w502, w505) -> (w519:cluster{dbl[], dbl[]})  [unwired: 1 in]
            n220 = Bundle(w502, w503) -> (w504:cluster{dbl[], dbl[]})  [unwired: 1 in]
            n221 = Build Array(w513, w514, w515, w516, w517, w518, w519, w504) -> (w512:cluster{dbl[], dbl[]}[])
          }
          frame "V, Keithley DAQ A4" {
            n222 = property on="MULTIPLE GRAPHS" class="XYGraph (strict)"("XScale.NameLbl.Text"="Keithley DAQ A4, V" ("X Scale.Name Label.Text")) -> ()  [unwired: 2 in, 2 out]
            n223 = Bundle(w530, w529) -> (w533:cluster{dbl[], dbl[]})  [unwired: 1 in]
            n224 = Bundle(w530, w528) -> (w534:cluster{dbl[], dbl[]})  [unwired: 1 in]
            n225 = Bundle(w530, w527) -> (w535:cluster{dbl[], dbl[]})  [unwired: 1 in]
            n226 = Bundle(w530, w526) -> (w536:cluster{dbl[], dbl[]})  [unwired: 1 in]
            n227 = Bundle(w530, w525) -> (w537:cluster{dbl[], dbl[]})  [unwired: 1 in]
            n228 = Bundle(w530, w524) -> (w538:cluster{dbl[], dbl[]})  [unwired: 1 in]
            n229 = Bundle(w530, w523) -> (w539:cluster{dbl[], dbl[]})  [unwired: 1 in]
            n230 = Bundle(w530, w522) -> (w532:cluster{dbl[], dbl[]})  [unwired: 1 in]
            n231 = Build Array(w533, w534, w535, w536, w537, w538, w539, w532) -> (w531:cluster{dbl[], dbl[]}[])
          }
          frame "V, Lock-In X" {
            n232 = property on="MULTIPLE GRAPHS" class="XYGraph (strict)"("XScale.NameLbl.Text"="Lock-In X, V" ("X Scale.Name Label.Text")) -> ()  [unwired: 2 in, 2 out]
            n233 = Bundle(w549, w548) -> (w551:cluster{dbl[], dbl[]})  [unwired: 1 in]
            n234 = Bundle(w549, w547) -> (w552:cluster{dbl[], dbl[]})  [unwired: 1 in]
            n235 = Bundle(w549, w546) -> (w553:cluster{dbl[], dbl[]})  [unwired: 1 in]
            n236 = Bundle(w549, w545) -> (w554:cluster{dbl[], dbl[]})  [unwired: 1 in]
            n237 = Bundle(w549, w544) -> (w555:cluster{dbl[], dbl[]})  [unwired: 1 in]
            n238 = Bundle(w549, w543) -> (w556:cluster{dbl[], dbl[]})  [unwired: 1 in]
            n239 = Bundle(w549, w542) -> (w557:cluster{dbl[], dbl[]})  [unwired: 1 in]
            n240 = Bundle(w549, w541) -> (w550:cluster{dbl[], dbl[]})  [unwired: 1 in]
            n241 = Build Array(w551, w552, w553, w554, w555, w556, w557, w550) -> (w540:cluster{dbl[], dbl[]}[])
          }
          frame "V, Lock-In Y" {
            n242 = property on="MULTIPLE GRAPHS" class="XYGraph (strict)"("XScale.NameLbl.Text"="Lock-In Y, V" ("X Scale.Name Label.Text")) -> ()  [unwired: 2 in, 2 out]
            n243 = Bundle(w568, w567) -> (w576:cluster{dbl[], dbl[]})  [unwired: 1 in]
            n244 = Bundle(w568, w566) -> (w575:cluster{dbl[], dbl[]})  [unwired: 1 in]
            n245 = Bundle(w568, w565) -> (w574:cluster{dbl[], dbl[]})  [unwired: 1 in]
            n246 = Bundle(w568, w564) -> (w573:cluster{dbl[], dbl[]})  [unwired: 1 in]
            n247 = Bundle(w568, w563) -> (w572:cluster{dbl[], dbl[]})  [unwired: 1 in]
            n248 = Bundle(w568, w562) -> (w571:cluster{dbl[], dbl[]})  [unwired: 1 in]
            n249 = Bundle(w568, w561) -> (w570:cluster{dbl[], dbl[]})  [unwired: 1 in]
            n250 = Bundle(w568, w560) -> (w569:cluster{dbl[], dbl[]})  [unwired: 1 in]
            n251 = Build Array(w576, w575, w574, w573, w572, w571, w570, w569) -> (w559:cluster{dbl[], dbl[]}[])
          }
        }
        "MULTIPLE GRAPHS" <- w222
        n252 = Unbundle(w231) -> (w254:dbl[], w253:dbl[], w252:dbl[], w251:dbl[], w250:dbl[], w249:dbl[], w184:dbl[], w185:dbl[], w186:dbl[], w187:dbl[])
        "2000" <- w386
        "DAQ A0" <- w204
        "DAQ A1" <- w203
        "DAQ A2" <- w202
        "DAQ A3" <- w201
        "DAQ A4" <- w194
      }
    }
    frame #3 {
      # "Closing instrumental \nconnections"
      n253 = Unbundle(w794) -> ("Task out"=w793:i32, "error out"=w792:errorcluster)
      n254 = call <instrlib>:"Close.vi"("VISA resource name"=w799, "error in (no error)"=w800) -> ()  [unwired: 17 in, 1 out]
      n255 = call "SR51XX Close"("error in (no error)"=w795, "VISA session"=w796) -> ()  [unwired: 1 out]
      n256 = call <instrlib>:"Close.vi"("VISA resource name"=w797, "error in (no error)"=w798) -> ()  [unwired: 13 in, 1 out]
      n257 = call <userlib>:"DtOLCloseTask.vi"("Error in"=w792, "Task in"=w793) -> ("Error Out"=w801:errorcluster)  [unwired: 9 in]
      n258 = call <vilib>:"Simple Error Handler.vi"("error in (no error)"=w801) -> ()  [unwired: 4 in, 5 out]
    }
  }
